vi "DetailedView.vi"(8 "error in (no error)":errorcluster, 10 "detailed":bool, 11 "TestView_Tree in":refnum<class "TestView_Tree_Single.lvclass">) -> (0 "error out":errorcluster, 3 "TestView_Tree out":refnum<class "TestView_Tree_Single.lvclass">)   [LabVIEW 2022 SP3, in "TestView_Tree_Single.lvlib" / "TestView_Tree_Single.lvclass"]
uses:
  TestView_Tree_Single.lvclass
  <vilib>/Utility/miscctls.llb/LVNodeAndColumnTypeDef.ctl
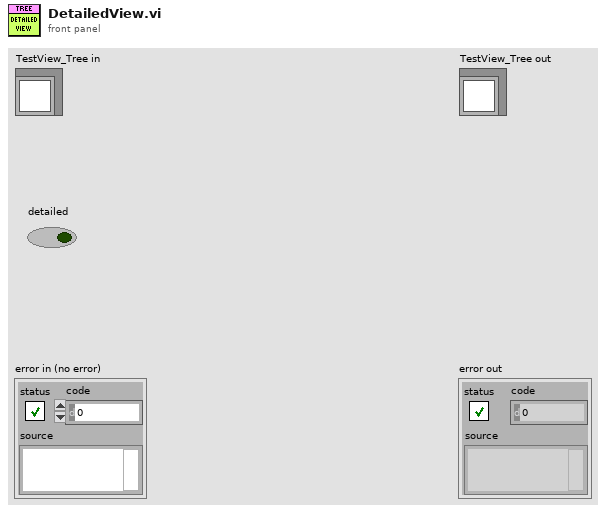
[diagram p1: front panel]
types:
  T1 = typedef "LVNodeAndColumnTypeDef.ctl" = cluster{"Node":string, "Column":i32}
  T2 = typedef "TestView_Tree_Single.lvlib/TestView_Tree_Single.lvclass/ObjectAttributes.ctl" = cluster{"Front Panel":refnum<vi>, "Last_Item":string, "Config":T3, "Title":string, "User":string, "TreeRef":refnum<vi>, "Active DUT":i32, "Status":T4, "SN":string, "Spec":string}
  T3 = typedef "TestView_Tree_Single.lvlib/TestView_Tree_Single.lvclass/Config.ctl" = cluster{"default":string}
  T4 = typedef "TestView_Base.lvlibp/TestView_Base.lvclass/ViewStatus.ctl" = enum16{"Testing", "Ready", "Logout", "Login", "PASS", "FAIL", "FAULT", "ABORTED"}
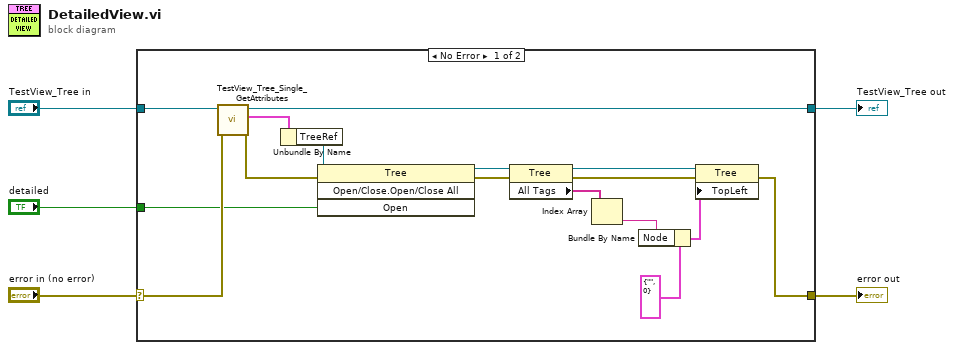
[diagram p0: block diagram]
diagram:
  n1 = case shown="No Error" "error in (no error)" {
    selector: "error in (no error)" -> [w19 w23]
    tunnel: [w14 w23] -> w4
    tunnel: [w20 w22] -> w2
    tunnel: "TestView_Tree in" -> [w21 w22]
    tunnel: "detailed" -> [w15 _]
    frame No Error {
      n2 = call "TestView_Tree_Single_GetAttributes.vi"("error in (no error)"=w19, "reference in"=w21) -> ("error out"=w16:errorcluster, "Data"=w18:T2, "reference out"=w20:refnum<class "TestView_Tree_Single.lvclass">)  [unwired: 6 in, 1 out]
      n3 = Unbundle By Name(w18) -> ("TreeRef"=w17:refnum<vi>)
      n4 = invoke class="Tree" method="Open/Close.Open/Close All"(reference=w17, error in=w16, "Open"=w15) -> (reference out=w11:refnum<vi>, error out=w13:errorcluster)  [unwired: 1 in, 2 out]
      n5 = property class="Tree"(reference=w11, error in=w13) -> (reference out=w10:refnum<vi>, error out=w12:errorcluster, "All Tags"=w9:string[])
      n6 = Index Array(array=w9) -> (element=w6:string)  [unwired: 1 in]
      n7 = Bundle By Name(cluster=T1 {"Node"="", "Column"=0} ("Top Left Visible Cell"), "Node"=w6) -> (w7:T1)
      n8 = property class="Tree"(reference=w10, error in=w12, "TopLeft"=w7) -> (error out=w14:errorcluster)  [unwired: 1 out]
    }
    frame Error {
    }
  }
  "error out" <- w4
  "TestView_Tree out" <- w2
